vi "TEST_DATA_3.vi"   [LabVIEW 2021]
uses:
  <vilib>/Utility/NIReport.llb/Report Type.ctl
  <vilib>/Utility/NIReport.llb/Append Text Table to Report (wrap).vi
  <vilib>/Utility/NIReport.llb/NI_report.lvclass
  <vilib>/Utility/NIReport.llb/NI_ReportGenerationCore.lvlib
types:
  T1 = typedef "NI_ReportGenerationCore.lvlib/Report Type.ctl" = enum16{"HTML", "Word", "Excel"}
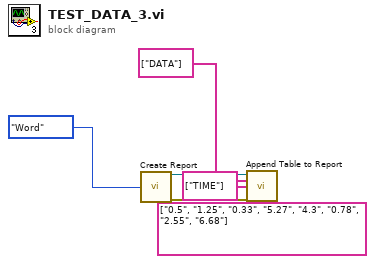
[diagram p0: block diagram]
diagram:
  n1 = call <vilib>:"Create Report.vi"("report type"=Report_Type."Word") -> ("report out"=w5:refnum<class "NI_report.lvclass">, "error out"=w4:errorcluster)  [unwired: 13 in]
  n2 = call-poly <vilib>:"Append Table to Report.vi"("report in"=w5, "column headers"=string[] ["DATA"], "row headers"=string[] ["TIME"], "text data"=string[][] [["0.5", "1.25", "0.33", "5.27"], ["4.3", "0.78", "2.55", "6.68"]], "error in (no error)"=w4) -> ()  [unwired: 7 in, 4 out]
